vi "Scale Point 3D (SGL) To Screen.vi"(7 "Screen Dimensions":T2, 11 "Point In":T1) -> (3 "Point Out":T1)   [LabVIEW 2020, in "3D (FPGA).lvlib"]
uses:
  3D (FPGA).lvlib
  Vector 3D.ctl
  Raster/Rectangle Dimensions.ctl
  Raster/Raster (FPGA).lvlib
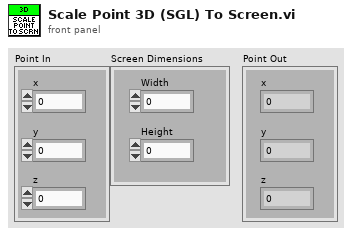
[diagram p1: front panel]
types:
  T1 = typedef "3D (FPGA).lvlib/Vector 3D.ctl" = cluster{"x":sgl, "y":sgl, "z":sgl}
  T2 = typedef "Raster (FPGA).lvlib/Rectangle Dimensions.ctl" = cluster{"Width":u32, "Height":u32}
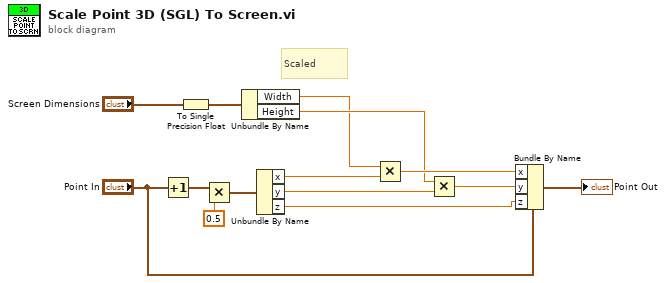
[diagram p0: block diagram]
diagram:
  # "Scaled"
  n1 = Increment(x="Point In") -> (x+1=w3:T1)
  n2 = To Single Precision Float(number="Screen Dimensions") -> (single precision float=w1:cluster{"Width":sgl, "Height":sgl})
  n3 = Multiply(x=w3, y=sgl 0.5 ("x")) -> (x*y=w5:T1)
  n4 = Unbundle By Name(w1) -> ("Width"=w8:sgl, "Height"=w10:sgl)
  n5 = Unbundle By Name(w5) -> ("x"=w7:sgl, "y"=w9:sgl, "z"=w13:sgl)
  n6 = Multiply(x=w8, y=w7) -> (x*y=w11:sgl)
  n7 = Multiply(x=w10, y=w9) -> (x*y=w12:sgl)
  n8 = Bundle By Name(cluster="Point In", "x"=w11, "y"=w12, "z"=w13) -> (→"Point Out":T1)
